vi "get cube parameters.vi"(4 "cnt":i32, 5 "Type":enum16{"Z", "I", "O", "S", "L", "J", "T", "N"}(ring)) -> (0 "angle":i8, 1 "c2":i8, 2 "c1":i8, 3 "level":i8)   [LabVIEW 2018]
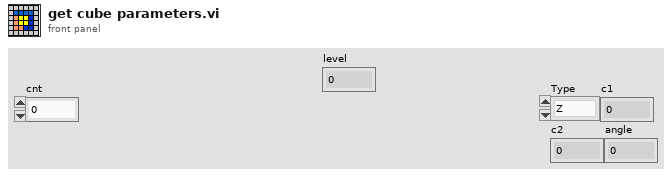
[diagram p1: front panel]
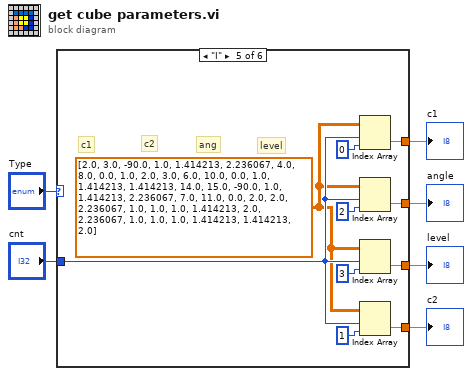
[diagram p0: block diagram]
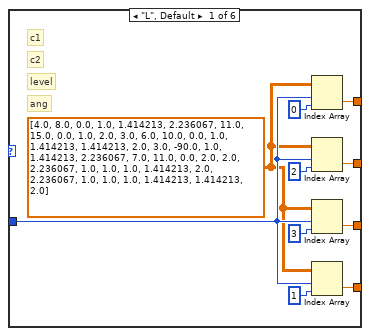
[diagram p2: hidden frame]
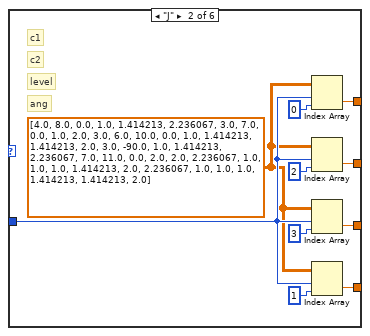
[diagram p3: hidden frame]
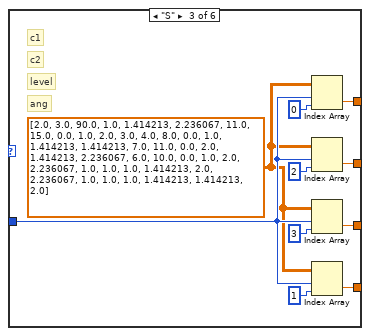
[diagram p4: hidden frame]
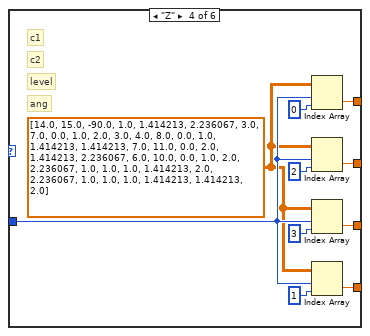
[diagram p5: hidden frame]
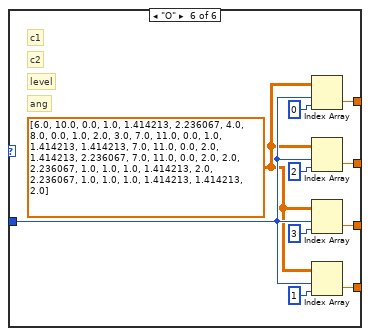
[diagram p6: hidden frame]
diagram:
  n1 = case shown="\"I\"" "Type" {
    tunnel: "cnt" -> [w9 w19 w29 w39 w49 w59]
    tunnel: [w15 w25 w35 w45 w55 w65] -> w4
    tunnel: [w13 w23 w33 w43 w53 w63] -> w3
    tunnel: [w11 w21 w31 w41 w51 w61] -> w2
    tunnel: [w7 w17 w27 w37 w47 w57] -> w1
    frame "L", Default {
      w8 = dbl[][] [[4.0, 8.0, 0.0, 1.0, 1.414213, 2.236067], [11.0, 15.0, 0.0, 1.0, 2.0, 3.0], [6.0, 10.0, 0.0, 1.0, 1.414213, 1.414213], [2.0, 3.0, -90.0, 1.0, 1.414213, 2.236067], [7.0, 11.0, 0.0, 2.0, 2.0, 2.236067], [1.0, 1.0, 1.0, 1.414213, 2.0, 2.236067], [1.0, 1.0, 1.0, 1.414213, 1.414213, 2.0]] ("Descriptors")
      # "level"
      # "ang"
      # "c2"
      # "c1"
      n2 = Index Array(array=w8, index (row)=w9, index (col)=0 ("disabled index (col)")) -> (element=w15:dbl)
      n3 = Index Array(array=w8, index (row)=w9, index (col)=2 ("disabled index (col)")) -> (element=w11:dbl)
      n4 = Index Array(array=w8, index (row)=w9, index (col)=3 ("disabled index (col)")) -> (element=w7:dbl)
      n5 = Index Array(array=w8, index (row)=w9, index (col)=1 ("disabled index (col)")) -> (element=w13:dbl)
    }
    frame "J" {
      w18 = dbl[][] [[4.0, 8.0, 0.0, 1.0, 1.414213, 2.236067], [3.0, 7.0, 0.0, 1.0, 2.0, 3.0], [6.0, 10.0, 0.0, 1.0, 1.414213, 1.414213], [2.0, 3.0, -90.0, 1.0, 1.414213, 2.236067], [7.0, 11.0, 0.0, 2.0, 2.0, 2.236067], [1.0, 1.0, 1.0, 1.414213, 2.0, 2.236067], [1.0, 1.0, 1.0, 1.414213, 1.414213, 2.0]] ("Descriptors")
      # "level"
      # "ang"
      # "c2"
      # "c1"
      n6 = Index Array(array=w18, index (row)=w19, index (col)=0 ("disabled index (col)")) -> (element=w25:dbl)
      n7 = Index Array(array=w18, index (row)=w19, index (col)=2 ("disabled index (col)")) -> (element=w21:dbl)
      n8 = Index Array(array=w18, index (row)=w19, index (col)=3 ("disabled index (col)")) -> (element=w17:dbl)
      n9 = Index Array(array=w18, index (row)=w19, index (col)=1 ("disabled index (col)")) -> (element=w23:dbl)
    }
    frame "S" {
      w28 = dbl[][] [[2.0, 3.0, 90.0, 1.0, 1.414213, 2.236067], [11.0, 15.0, 0.0, 1.0, 2.0, 3.0], [4.0, 8.0, 0.0, 1.0, 1.414213, 1.414213], [7.0, 11.0, 0.0, 2.0, 1.414213, 2.236067], [6.0, 10.0, 0.0, 1.0, 2.0, 2.236067], [1.0, 1.0, 1.0, 1.414213, 2.0, 2.236067], [1.0, 1.0, 1.0, 1.414213, 1.414213, 2.0]] ("Descriptors")
      # "level"
      # "ang"
      # "c2"
      # "c1"
      n10 = Index Array(array=w28, index (row)=w29, index (col)=0 ("disabled index (col)")) -> (element=w35:dbl)
      n11 = Index Array(array=w28, index (row)=w29, index (col)=2 ("disabled index (col)")) -> (element=w31:dbl)
      n12 = Index Array(array=w28, index (row)=w29, index (col)=3 ("disabled index (col)")) -> (element=w27:dbl)
      n13 = Index Array(array=w28, index (row)=w29, index (col)=1 ("disabled index (col)")) -> (element=w33:dbl)
    }
    frame "Z" {
      w38 = dbl[][] [[14.0, 15.0, -90.0, 1.0, 1.414213, 2.236067], [3.0, 7.0, 0.0, 1.0, 2.0, 3.0], [4.0, 8.0, 0.0, 1.0, 1.414213, 1.414213], [7.0, 11.0, 0.0, 2.0, 1.414213, 2.236067], [6.0, 10.0, 0.0, 1.0, 2.0, 2.236067], [1.0, 1.0, 1.0, 1.414213, 2.0, 2.236067], [1.0, 1.0, 1.0, 1.414213, 1.414213, 2.0]] ("Descriptors")
      # "level"
      # "ang"
      # "c2"
      # "c1"
      n14 = Index Array(array=w38, index (row)=w39, index (col)=0 ("disabled index (col)")) -> (element=w45:dbl)
      n15 = Index Array(array=w38, index (row)=w39, index (col)=2 ("disabled index (col)")) -> (element=w41:dbl)
      n16 = Index Array(array=w38, index (row)=w39, index (col)=3 ("disabled index (col)")) -> (element=w37:dbl)
      n17 = Index Array(array=w38, index (row)=w39, index (col)=1 ("disabled index (col)")) -> (element=w43:dbl)
    }
    frame "I" {
      w48 = dbl[][] [[2.0, 3.0, -90.0, 1.0, 1.414213, 2.236067], [4.0, 8.0, 0.0, 1.0, 2.0, 3.0], [6.0, 10.0, 0.0, 1.0, 1.414213, 1.414213], [14.0, 15.0, -90.0, 1.0, 1.414213, 2.236067], [7.0, 11.0, 0.0, 2.0, 2.0, 2.236067], [1.0, 1.0, 1.0, 1.414213, 2.0, 2.236067], [1.0, 1.0, 1.0, 1.414213, 1.414213, 2.0]] ("Descriptors")
      # "level"
      # "ang"
      # "c2"
      # "c1"
      n18 = Index Array(array=w48, index (row)=w49, index (col)=0 ("disabled index (col)")) -> (element=w55:dbl)
      n19 = Index Array(array=w48, index (row)=w49, index (col)=2 ("disabled index (col)")) -> (element=w51:dbl)
      n20 = Index Array(array=w48, index (row)=w49, index (col)=3 ("disabled index (col)")) -> (element=w47:dbl)
      n21 = Index Array(array=w48, index (row)=w49, index (col)=1 ("disabled index (col)")) -> (element=w53:dbl)
    }
    frame "O" {
      w58 = dbl[][] [[6.0, 10.0, 0.0, 1.0, 1.414213, 2.236067], [4.0, 8.0, 0.0, 1.0, 2.0, 3.0], [7.0, 11.0, 0.0, 1.0, 1.414213, 1.414213], [7.0, 11.0, 0.0, 2.0, 1.414213, 2.236067], [7.0, 11.0, 0.0, 2.0, 2.0, 2.236067], [1.0, 1.0, 1.0, 1.414213, 2.0, 2.236067], [1.0, 1.0, 1.0, 1.414213, 1.414213, 2.0]] ("Descriptors")
      # "level"
      # "ang"
      # "c2"
      # "c1"
      n22 = Index Array(array=w58, index (row)=w59, index (col)=0 ("disabled index (col)")) -> (element=w65:dbl)
      n23 = Index Array(array=w58, index (row)=w59, index (col)=2 ("disabled index (col)")) -> (element=w61:dbl)
      n24 = Index Array(array=w58, index (row)=w59, index (col)=3 ("disabled index (col)")) -> (element=w57:dbl)
      n25 = Index Array(array=w58, index (row)=w59, index (col)=1 ("disabled index (col)")) -> (element=w63:dbl)
    }
  }
  "c1" <- w4
  "c2" <- w3
  "angle" <- w2
  "level" <- w1
